vi "GPS Give Heading.vi"(2 "Target Position":cluster{"Latitude":dbl, "Longitude":dbl}, 3 "Current State":T1) -> (0 "Wheel Angle":i8, 1 "Target Heading":dbl)   [LabVIEW 2009]
panel:
  # "Latitude are on a x- and y-coordinates,\nE is +x, and N is +y.  Heading is different:\nN is 0 deg, and increases clock-wise.  E is\n90, S is 180 and W is 270."
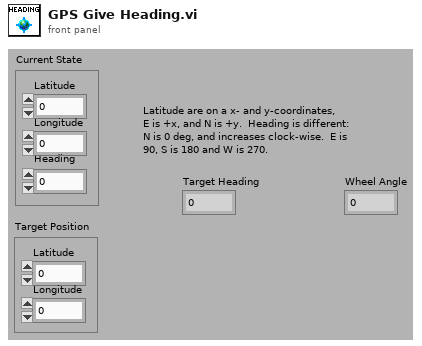
[diagram p1: front panel]
types:
  T1 = cluster{"Latitude":dbl, "Heading":dbl, "Longitude":dbl}
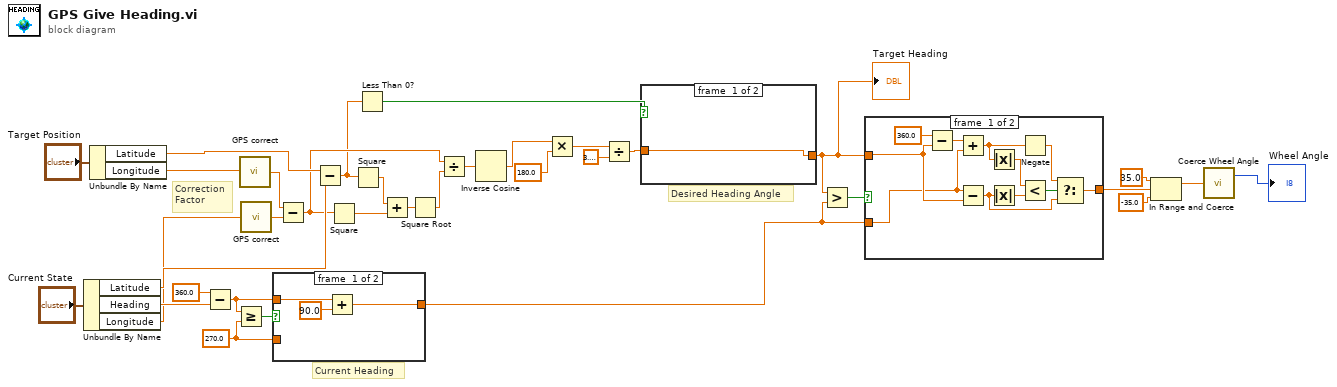
[diagram p0: block diagram]
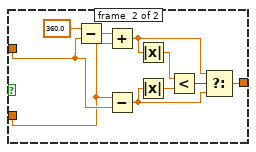
[diagram p2: hidden frame]
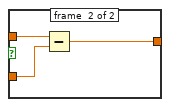
[diagram p3: hidden frame]
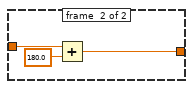
[diagram p4: hidden frame]
diagram:
  w15 = 270.0 ("y")
  # "Correction\nFactor"
  # "Current Heading"
  # "Desired Heading Angle"
  n1 = Unbundle By Name("Current State") -> ("Latitude"=w32:dbl, "Heading"=w19:dbl, "Longitude"=w6:dbl)
  n2 = Unbundle By Name("Target Position") -> ("Latitude"=w27:dbl, "Longitude"=w3:dbl)
  n3 = Subtract(x=360.0, y=w19) -> (x-y=w16:dbl)
  n4 = Greater Or Equal?(x=w16, y=w15) -> (x >= y?=w17:bool)
  n5 = call "GPS correct.vi"("Raw Longitude"=w3) -> ("Corrected Longitude"=w4:dbl)
  n6 = call "GPS correct.vi"("Raw Longitude"=w6) -> ("Corrected Longitude"=w5:dbl)
  n7 = case shown="True" w17 {
    tunnel: w16 -> [w37 w40]
    tunnel: w15 -> [_ w39]
    tunnel: [w35 w38] -> w12
    frame #0 {
      n8 = Add(x=w37, y=90.0) -> (x+y=w35:dbl)
    }
    frame #1 {
      n9 = Subtract(x=w40, y=w39) -> (x-y=w38:dbl)
    }
  }
  n10 = Subtract(x=w4, y=w5) -> (x-y=w2:dbl)
  n11 = Subtract(x=w27, y=w32) -> (x-y=w1:dbl)
  n12 = Square(x=w2) -> (x^2=w29:dbl)
  n13 = Square(x=w1) -> (x^2=w30:dbl)
  n14 = Less Than 0?(x=w1) -> (x < 0?=w25:bool)
  n15 = Add(x=w30, y=w29) -> (x+y=w31:dbl)
  n16 = Square Root(x=w31) -> (sqrt(x)=w28:dbl)
  n17 = Divide(x=w2, y=w28) -> (x/y=w26:dbl)
  n18 = Inverse Cosine(1:w26) -> (0:w24:dbl)
  n19 = Multiply(x=w24, y=180.0) -> (x*y=w23:dbl)
  n20 = Divide(x=w23, y=3.141592653589793) -> (x/y=w22:dbl)
  n21 = case shown="False" w25 {
    tunnel: w22 -> [w41 w44]
    tunnel: [w41 w42] -> w13
    frame #0 {
    }
    frame #1 {
      n22 = Add(x=w44, y=180.0) -> (x+y=w42:dbl)
    }
  }
  "Target Heading" <- w13
  n23 = Greater?(x=w13, y=w12) -> (0:w14:bool)
  n24 = case shown="True" w14 {
    tunnel: w13 -> [w49 w63]
    tunnel: w12 -> [w48 w62]
    tunnel: [w45 w56] -> w11
    frame #0 {
      n25 = Subtract(x=360.0, y=w49) -> (x-y=w51:dbl)
      n26 = Add(x=w51, y=w48) -> (x+y=w46:dbl)
      n27 = Subtract(x=w48, y=w49) -> (x-y=w55:dbl)
      n28 = Absolute Value(x=w46) -> (abs(x)=w52:dbl)
      n29 = Absolute Value(x=w55) -> (abs(x)=w53:dbl)
      n30 = Negate(x=w46) -> (-x=w47:dbl)
      n31 = Less?(x=w52, y=w53) -> (x < y?=w54:bool)
      n32 = Select(t=w47, s=w54, f=w55) -> (s? t:f=w45:dbl)
    }
    frame #1 {
      n33 = Subtract(x=360.0, y=w63) -> (x-y=w64:dbl)
      n34 = Add(x=w64, y=w62) -> (x+y=w58:dbl)
      n35 = Subtract(x=w62, y=w63) -> (x-y=w57:dbl)
      n36 = Absolute Value(x=w58) -> (abs(x)=w61:dbl)
      n37 = Absolute Value(x=w57) -> (abs(x)=w60:dbl)
      n38 = Less?(x=w61, y=w60) -> (x < y?=w59:bool)
      n39 = Select(t=w58, s=w59, f=w57) -> (s? t:f=w56:dbl)
    }
  }
  n40 = In Range and Coerce(upper limit=35.0, x=w11, lower limit=-35.0) -> (coerced(x)=w8:dbl)  [unwired: 1 out]
  n41 = call "Coerce Wheel Angle.vi"("Angle In"=w8) -> ("Wheel Angle"=→"Wheel Angle":i8)  [unwired: 1 out]
